vi "Read Record Data.vi"(8 "Error In (no error)":errorcluster, 11 "Expenses Tracker Balance In":refnum<class "Expenses Tracker Balance.lvclass">) -> (0 "Error Out":errorcluster, 2 "Record":variant, 3 "Expenses Tracker Balance Out":refnum<class "Expenses Tracker Balance.lvclass">)   [LabVIEW 2023, in "Expenses Tracker Balance.lvclass"]
uses:
  Expenses Tracker Balance.lvclass
  Expenses Tracker Balance.lvclass/Expenses Tracker Balance.ctl
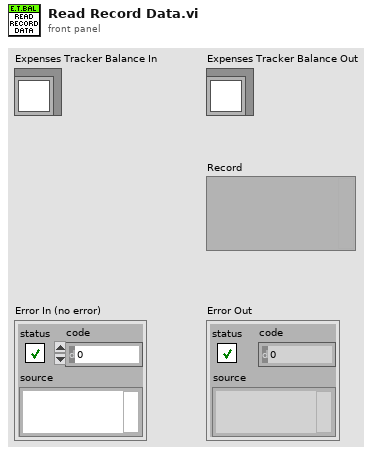
[diagram p1: front panel]
types:
  T1 = typedef "Expenses Tracker Balance.lvclass/Balance.ctl" = cluster{"ID":u8, "Value":dbl, "Last_update":timestamp}
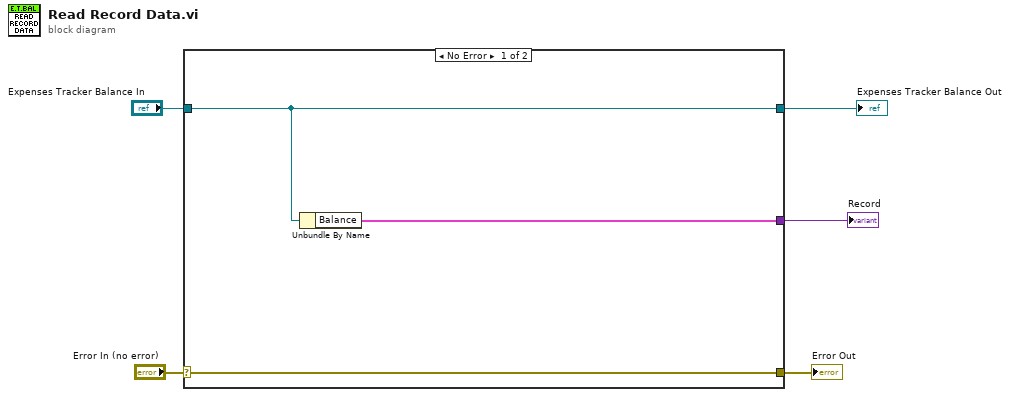
[diagram p0: block diagram]
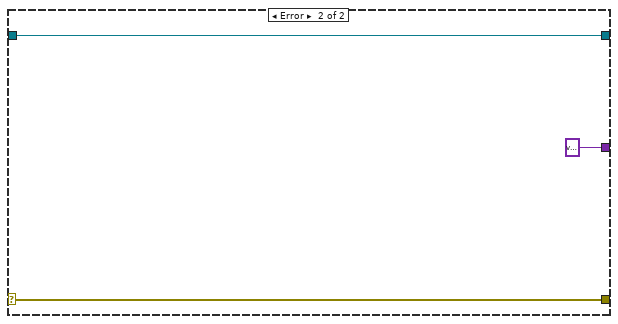
[diagram p2: hidden frame]
diagram:
  n1 = case shown="No Error" "Error In (no error)" {
    selector: "Error In (no error)" -> [w8 w11]
    tunnel: [w8 w11] -> w2
    tunnel: [w7 w10] -> w5
    tunnel: "Expenses Tracker Balance In" -> [w7 w10]
    tunnel: [w6 variant] -> w1
    frame No Error {
      n2 = Unbundle By Name(w7) -> ("Balance"=w6:T1)
    }
    frame Error {
    }
  }
  "Error Out" <- w2
  "Expenses Tracker Balance Out" <- w5
  "Record" <- w1
